vi "Inputs_DriverStation.vi"() -> ()   [LabVIEW 2018]
panel:
  in  "ButterflyState":bool
  out "Y Joystick":dbl
  out "X Joystick":dbl
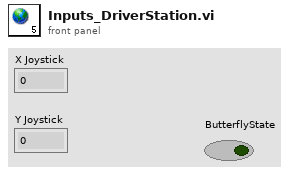
[diagram p1: front panel]
diagram:
